vi "Crop Image.vi"(10 "Cropped Image":T1, 11 "Camera Image":T1) -> (2 "Y Resolution":i32, 3 "Cropped Image":T1, 4 "X Resolution":i32)   [LabVIEW 2012]
uses:
  <vilib>/vision/Image Controls.llb/IMAQ Image.ctl
  <vilib>/vision/NI_Vision_Development_Module.lvlib
panel:
  in  "Botom Percent":dbl=0.45
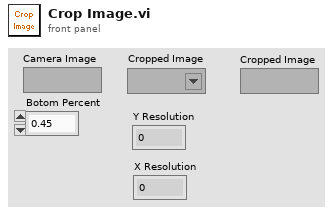
[diagram p1: front panel]
types:
  T1 = typedef "IMAQ Image.ctl" = refnum<image>
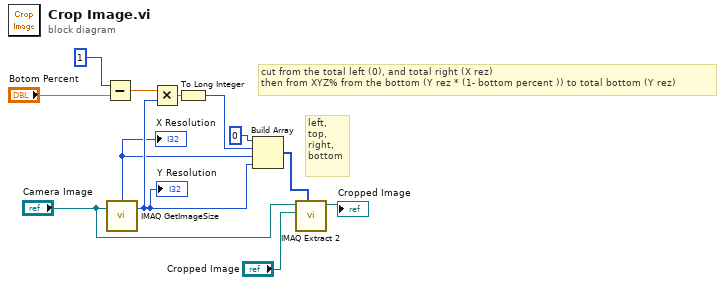
[diagram p0: block diagram]
diagram:
  # "cut from the total left (0), and total right (X rez)\nthen from XYZ% from the bottom (Y rez * (1- bottom percent )) to total bottom (Y rez)"
  # "left, \ntop, \nright, \nbottom"
  n1 = Subtract(x=1, y="Botom Percent") -> (x-y=w9:dbl)
  n2 = call "IMAQ GetImageSize"("Image"="Camera Image") -> ("Y Resolution"=w2:i32, "X Resolution"=w1:i32)  [unwired: 3 in, 1 out]
  "Y Resolution" <- w2
  "X Resolution" <- w1
  n3 = Multiply(x=w9, y=w2) -> (x*y=w6:dbl)
  n4 = To Long Integer(number=w6) -> (32bit integer=w8:i32)
  n5 = Build Array(0, w8, w1, w2) -> (w7:i32[])
  n6 = call "IMAQ Extract 2"("Optional Rectangle"=w7, "Image Dst"="Cropped Image", "Image Src"="Camera Image") -> ("Image Dst Out"=→"Cropped Image":T1)  [unwired: 7 in, 1 out]
